vi "sinanju_move.vi"(0 "VISA资源名称":refnum<visa-resource-name>, 1 "y1":sgl, 2 "h1":sgl, 3 "y1 2":sgl, 4 "h1 2":sgl, 5 "ax":i32, 6 "t":sgl, 7 "page":i32, 8 "错误输入（无错误）":errorcluster, 9 "mode":i32, 11 "x1":sgl, 12 "z1":sgl, 13 "x1 2":sgl, 14 "z1 2":sgl) -> (10 "VISA资源名称输出":refnum<visa-resource-name>, 15 "错误输出":errorcluster)   [LabVIEW 2017]
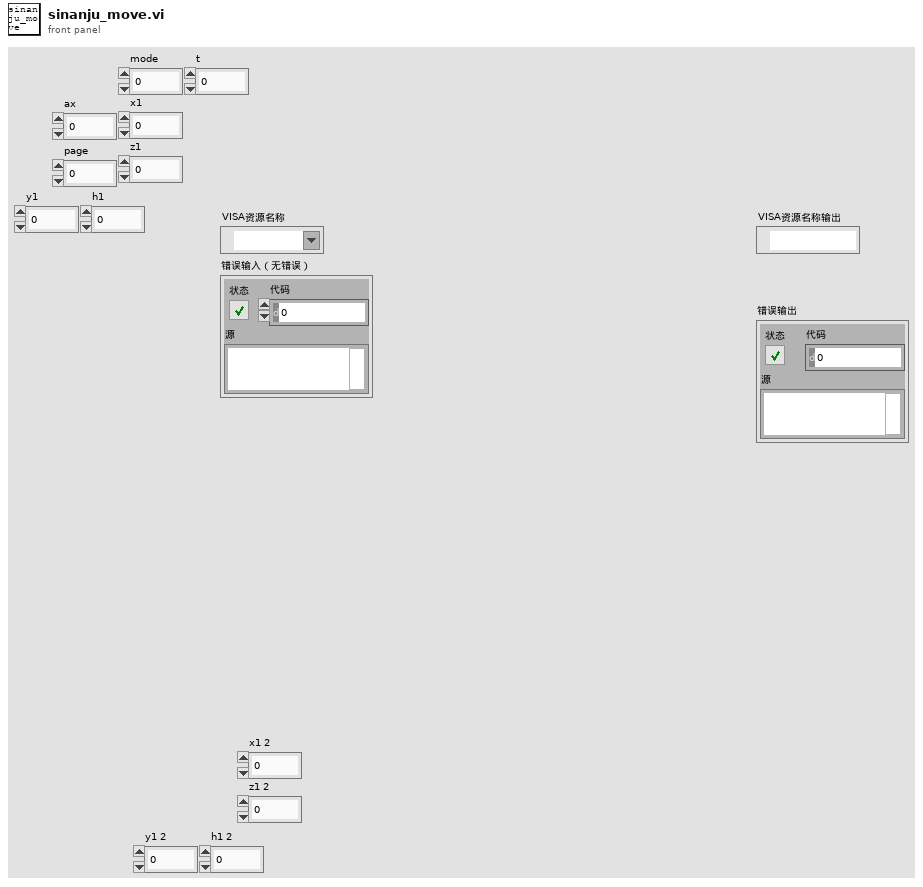
[diagram p1: front panel]
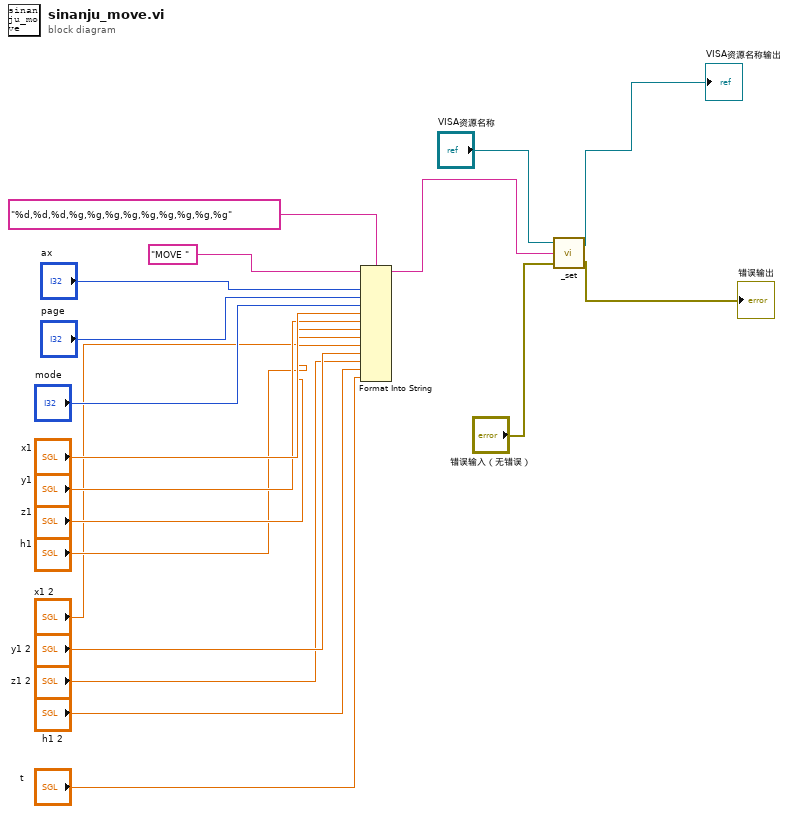
[diagram p0: block diagram]
diagram:
  n1 = Format Into String(format string="%d,%d,%d,%g,%g,%g,%g,%g,%g,%g,%g,%g" ("格式字符串"), initial string="MOVE " ("初始字符串"), "ax", "page", "mode", "x1", "y1", "z1", "h1", "x1 2", "y1 2", "z1 2", "h1 2", "t") -> (resulting string=w14:string)  [unwired: 1 in, 1 out]
  n2 = call "_set.vi"("错误输入（无错误）"="错误输入（无错误）", "写入缓冲区"=w14, "VISA资源名称输出 2"="VISA资源名称") -> ("错误输出"=→"错误输出":errorcluster, "VISA资源名称输出"=→"VISA资源名称输出":refnum<visa-resource-name>)
